vi "Power Status Display.vi"(0 "MSI Data":T1 {"Converter Faults 2" format="%016b"; "Converter Alarms 2" format="%016b"; "Converter Faults 1" format="%016b"; "Converter Alarms 1" format="%016b"; "Solar Faults" format="%016b"; "ES Rack 10 Alarms" format="%016b"; "ES Rack 9 Alarms" format="%016b"; "ES Rack 8 Alarms" format="%016b"; "ES Rack 7 Alarms" format="%016b"; "ES Rack 6 Alarms" format="%016b"; "ES Rack 5 Alarms" format="%016b"; "ES Rack 4 Alarms" format="%016b"; "ES Rack 3 Alarms" format="%016b"; "ES Rack 2 Alarms" format="%016b"; "ES Rack 1 Alarms" format="%016b"; "ES System Alarms" format="%016b"; "System Faults" format="%016b"; "ES Rack 10 Faults" format="%016b"; "Es Rack 9 Faults" format="%016b"; "ES Rack 8 Faults" format="%016b"; "ES Rack 7 Faults" format="%016b"; "ES Rack 6 Faults" format="%016b"; "ES Rack 5 Faults" format="%016b"; "ES Rack 4 Faults" format="%016b"; "ES Rack 3 Faults" format="%016b"; "ES Rack 2 Faults" format="%016b"; "ES Rack 1 Faults" format="%016b"; "ES System Faults" format="%016b"; "System Status" format="%016b"; "Controller Faults" format="%016b"}, 3 "Connection Error":bool, 11 "Error In":errorcluster) -> (6 "System Status Data":bool[](array[boolean]), 8 "Gen Status Data":bool[](array[boolean]), 13 "Status Select":u16, 15 "Error Out":errorcluster)   [LabVIEW 2014]
uses:
  Controls/Modbus Status Interface Data MOD2.ctl
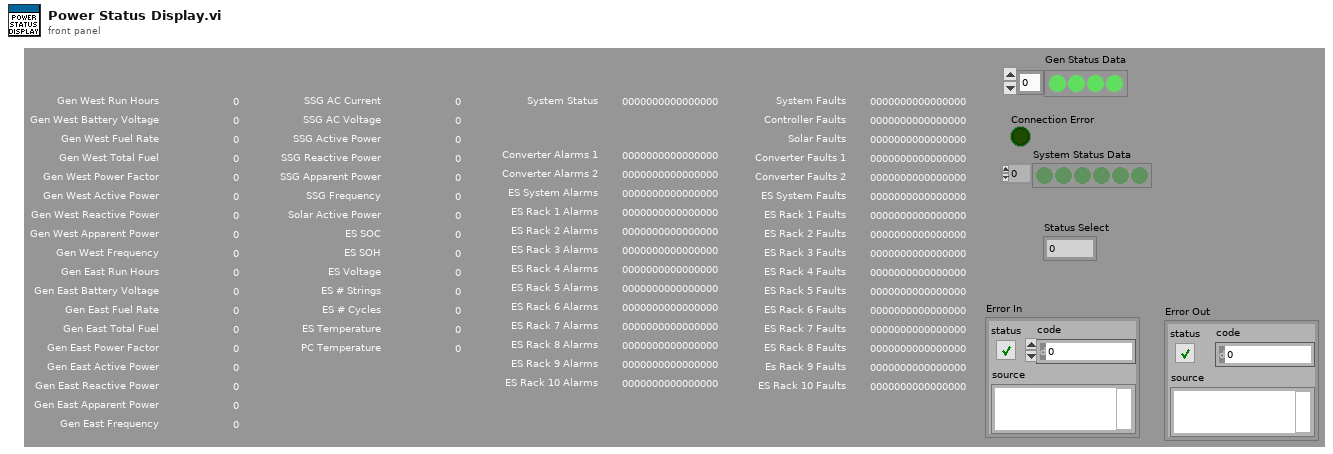
[diagram p1: front panel]
types:
  T1 = typedef "Modbus Status Interface Data MOD2.ctl" = cluster{"SSG AC Current":i16, "SSG AC Voltage":i16, "SSG Active Power":i16, "SSG Reactive Power":i16, "SSG Apparent Power":i16, "SSG Frequency":i16, "ES SOC":i16, "ES SOH":i16, "ES Voltage":i16, "ES # Strings":i16, "ES # Cycles":i16, "ES Temperature":i16, "PC Temperature":i16, "Solar Active Power":i16, "Gen West Run Hours":i16, "Gen West Battery Voltage":i16, "Gen West Fuel Rate":i16, "Gen West Total Fuel":i16, "Gen West Power Factor":i16, "Gen West Active Power":i16, "Gen West Reactive Power":i16, "Gen West Apparent Power":i16, "Gen West Frequency":i16, "Gen East Run Hours":i16, "Gen East Battery Voltage":i16, "Gen East Fuel Rate":i16, "Gen East Total Fuel":i16, "Gen East Power Factor":i16, "Gen East Active Power":i16, "Gen East Reactive Power":i16, "Gen East Apparent Power":i16, "Gen East Frequency":i16, "Converter Version":i16, "Controller Version":i16, "System Status":i16, "System Faults":i16, "Controller Faults":i16, "ES System Faults":i16, "ES System Alarms":i16, "Converter Faults 1":i16, "Converter Faults 2":i16, "Converter Alarms 1":i16, "Converter Alarms 2":i16, "Solar Faults":i16, "ES Rack 1 Faults":i16, "ES Rack 2 Faults":i16, "ES Rack 3 Faults":i16, "ES Rack 4 Faults":i16, "ES Rack 5 Faults":i16, "ES Rack 6 Faults":i16, "ES Rack 7 Faults":i16, "ES Rack 8 Faults":i16, "Es Rack 9 Faults":i16, "ES Rack 10 Faults":i16, "ES Rack 1 Alarms":i16, "ES Rack 2 Alarms":i16, "ES Rack 3 Alarms":i16, "ES Rack 4 Alarms":i16, "ES Rack 5 Alarms":i16, "ES Rack 6 Alarms":i16, "ES Rack 7 Alarms":i16, "ES Rack 8 Alarms":i16, "ES Rack 9 Alarms":i16, "ES Rack 10 Alarms":i16}
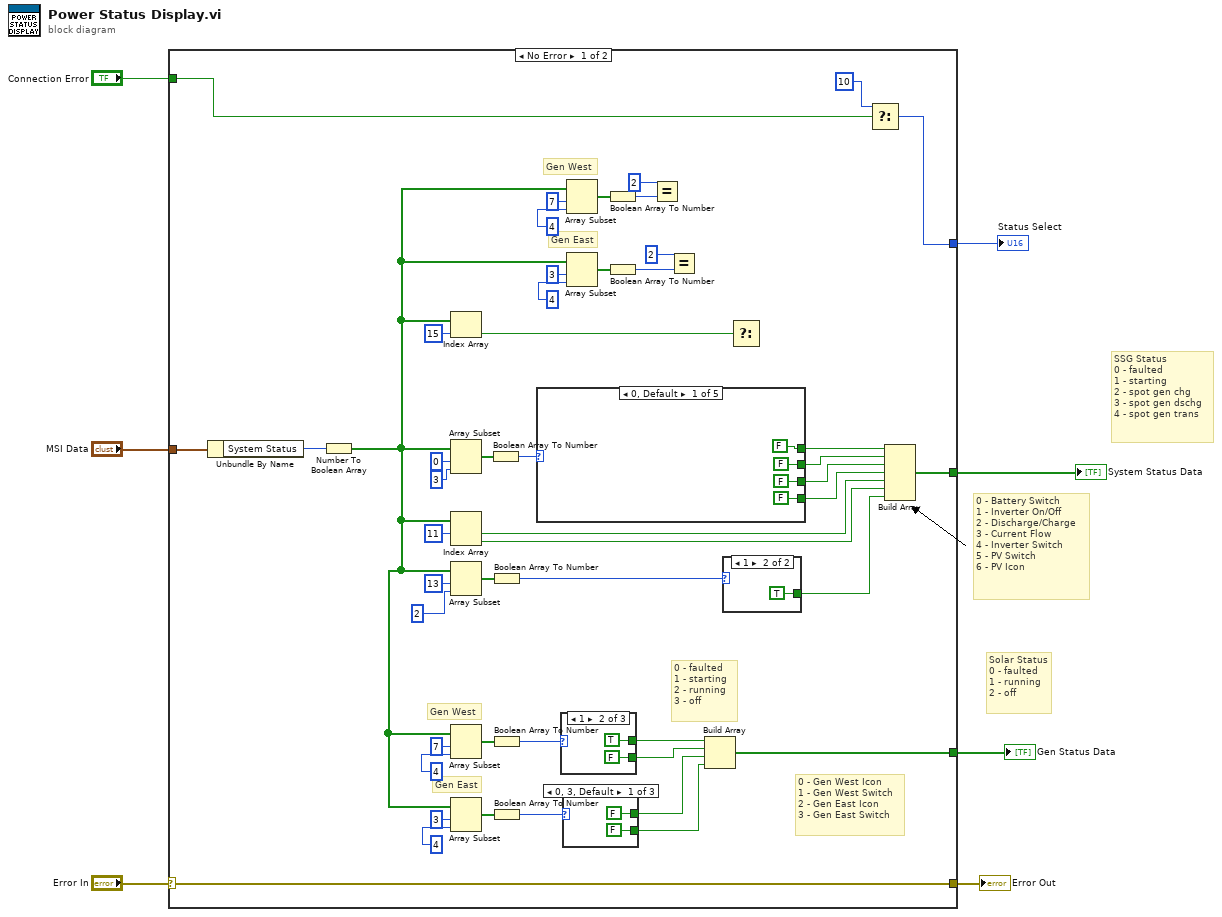
[diagram p0: block diagram]
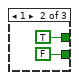
[diagram p2: hidden frame]
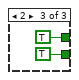
[diagram p3: hidden frame]
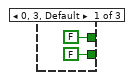
[diagram p4: hidden frame]
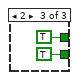
[diagram p5: hidden frame]
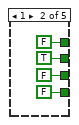
[diagram p6: hidden frame]
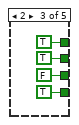
[diagram p7: hidden frame]
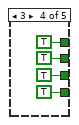
[diagram p8: hidden frame]
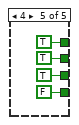
[diagram p9: hidden frame]
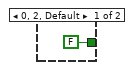
[diagram p10: hidden frame]
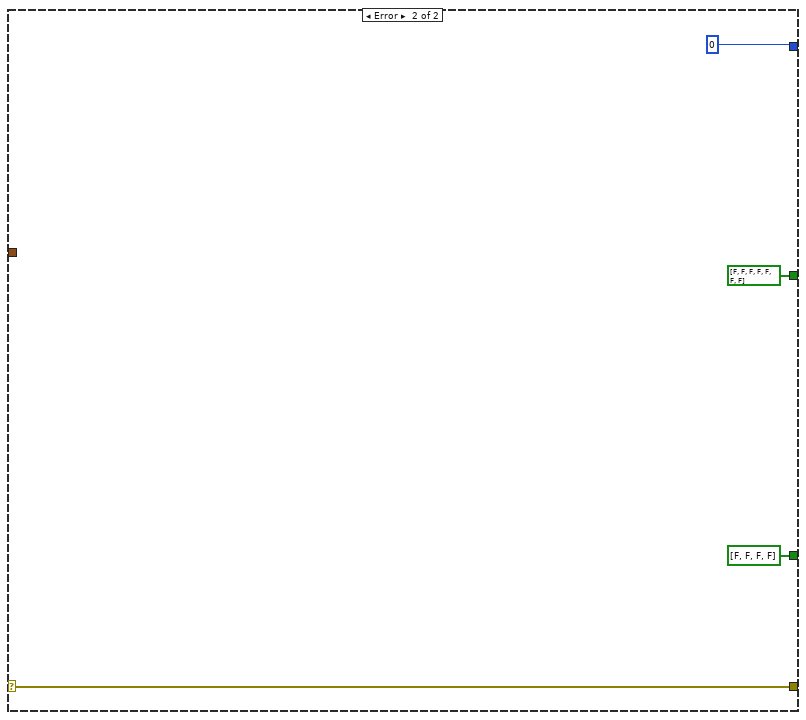
[diagram p11: hidden frame]
diagram:
  # "0 - Battery Switch\n1 - Inverter On/Off\n2 - Discharge/Charge\n3 - Current Flow\n4 - Inverter Switch\n5 - PV Switch\n6 - PV Icon"
  # "Solar Status\n0 - faulted\n1 - running\n2 - off"
  # "SSG Status\n0 - faulted\n1 - starting\n2 - spot gen chg\n3 - spot gen dschg\n4 - spot gen trans"
  n1 = case shown="No Error" "Error In" {
    selector: "Error In" -> [w49 w94]
    tunnel: [w49 w94] -> w6
    tunnel: "MSI Data" -> [w56 _]
    tunnel: "Connection Error" -> [w20 _]
    tunnel: [w35 bool[] [FALSE, FALSE, FALSE, FALSE]] -> w3
    tunnel: [w27 bool[] [FALSE, FALSE, FALSE, FALSE, FALSE, FALSE, FALSE]] -> w2
    tunnel: [w21 u16 0] -> w1
    frame No Error {
      # "Gen East"
      # "Gen West"
      # "Gen East"
      # "Gen West"
      # "0 - Gen West Icon\n1 - Gen West Switch\n2 - Gen East Icon\n3 - Gen East Switch"
      # "0 - faulted\n1 - starting\n2 - running \n3 - off"
      n2 = Unbundle By Name(w56) -> ("System Status"=w55:i16)
      n3 = Number To Boolean Array(number=w55) -> (Boolean array=w14:bool[])
      n4 = Index Array(array=w14, index=15) -> (element=w23:bool)
      n5 = Array Subset(array=w14, index=0, length=3) -> (w26:bool[])
      n6 = Index Array(array=w14, index #1=11 ("index")) -> (element #1=w30:bool, element #2=w29:bool)  [unwired: 1 in]
      n7 = Array Subset(array=w14, index=13, length=2 ("index")) -> (w50:bool[])
      n8 = Array Subset(array=w14, index=7, length=4) -> (w41:bool[])
      n9 = Array Subset(array=w14, index=3, length=4) -> (w38:bool[])
      n10 = Boolean Array To Number(Boolean array=w26) -> (number=w25:u32)
      n11 = Boolean Array To Number(Boolean array=w50) -> (number=w24:u32)
      n12 = Boolean Array To Number(Boolean array=w41) -> (number=w37:u8)
      n13 = Boolean Array To Number(Boolean array=w38) -> (number=w36:u8)
      n14 = case shown="0, Default" w25 {
        tunnel: [FALSE TRUE TRUE TRUE TRUE] -> w33
        tunnel: [FALSE FALSE FALSE TRUE TRUE] -> w32
        tunnel: [FALSE FALSE TRUE TRUE FALSE] -> w31
        tunnel: [FALSE FALSE TRUE TRUE TRUE] -> w34
        frame 0, Default {
        }
        frame 1 {
        }
        frame 2 {
        }
        frame 3 {
        }
        frame 4 {
        }
      }
      n15 = case shown="1" w37 {
        tunnel: [FALSE TRUE TRUE] -> w47
        tunnel: [FALSE FALSE TRUE] -> w46
        frame 0, 3, Default {
        }
        frame 1 {
        }
        frame 2 {
        }
      }
      n16 = case shown="0, 3, Default" w36 {
        tunnel: [FALSE TRUE TRUE] -> w45
        tunnel: [FALSE FALSE TRUE] -> w44
        frame 0, 3, Default {
        }
        frame 1 {
        }
        frame 2 {
        }
      }
      n17 = Array Subset(array=w14, index=7, length=4) -> (w13:bool[])
      n18 = Array Subset(array=w14, index=3, length=4) -> (w12:bool[])
      n19 = Boolean Array To Number(Boolean array=w13) -> (number=w11:u8)
      n20 = Boolean Array To Number(Boolean array=w12) -> (number=w8:u8)
      n21 = Equal?(x=u8 2, y=w11) -> ()  [unwired: 1 out]
      n22 = Equal?(x=u8 2, y=w8) -> ()  [unwired: 1 out]
      n23 = Build Array(w47, w46, w45, w44) -> (w35:bool[])
      n24 = case shown="1" w24 {
        tunnel: [FALSE TRUE] -> w28
        frame 0, 2, Default {
        }
        frame 1 {
        }
      }
      n25 = Select(s=w23) -> ()  [unwired: 2 in, 1 out]
      n26 = Select(t=u16 10, s=w20) -> (s? t:f=w21:u16)  [unwired: 1 in]
      n27 = Build Array(w34, w33, w32, w31, w30, w29, w28) -> (w27:bool[])
    }
    frame Error {
    }
  }
  "Error Out" <- w6
  "System Status Data" <- w2
  "Gen Status Data" <- w3
  "Status Select" <- w1
